vi "pp2_stateToDOCode.vi"(11 "State In":T1={"Curr  tr"=0, "Curr (ms)"=0, "Cum (ms)"=0, "Run loop diff"=0, "Curr State"=enum."0 Initialization", "Prev State"=enum."0 Initialization", "Sw1"=FALSE, "Tone Gate"=FALSE, "Stim"=FALSE, "Sw2"=FALSE, "Curr code"=0, "Current Trial"={"Trial Type Number"=1, "Trial Type"=enum."GO", "Trial Weight"=100, "Shock (mA)"=0.3, "Duration (ms)"=0.25, "Type"=enum."04 FM Sweep", "Stim P2"=4000.0, "Stim P3"=0.0, "Stim P4"=0.0, "Stim P1"=2000.0}, "Last tone"=0, "Countdown (ms)"=0, "Next Trial"={"Trial Type Number"=1, "Trial Type"=enum."GO", "Trial Weight"=100, "Shock (mA)"=0.3, "Duration (ms)"=0.25, "Type"=enum."04 FM Sweep", "Stim P2"=4000.0, "Stim P3"=0.0, "Stim P4"=0.0, "Stim P1"=2000.0}, "Current DAQ Digital Out"=0} {"Current DAQ Digital Out" format="%b"; "Next Trial"."Shock (mA)" min=-1.0 max=5.0; "Next Trial"."Trial Weight" step=1; "Next Trial"."Duration (ms)" min=0.0 max=1.0; "Next Trial"."Trial Type Number" min=1 max=256 step=1; "Current Trial"."Shock (mA)" min=-1.0 max=5.0; "Current Trial"."Trial Weight" step=1; "Current Trial"."Duration (ms)" min=0.0 max=1.0; "Current Trial"."Trial Type Number" min=1 max=256 step=1; "Curr code" format="%#.6f"}) -> (3 "DAQ Digital Code":u16 format="%b")   [LabVIEW 2013]
uses:
  pp2_CTL_StateInfo.ctl
  pp2_State.ctl
  pp2_Trial.ctl
  pp2_TrialType.ctl
  labolabo2/waveforms/WFTypes.ctl
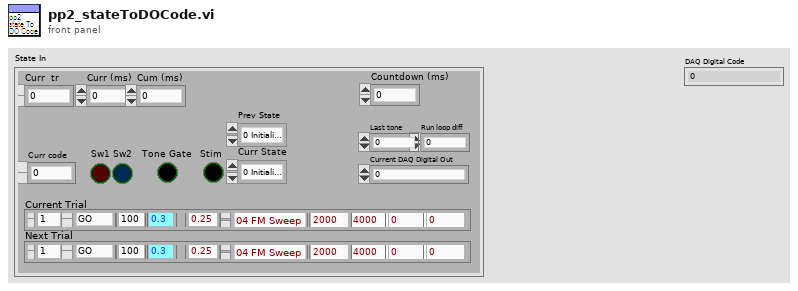
[diagram p1: front panel]
types:
  T1 = typedef "pp2_CTL_StateInfo.ctl" = cluster{"Curr  tr":u16, "Curr (ms)":i64, "Cum (ms)":i64, "Run loop diff":i64, "Curr State":T2, "Prev State":T2, "Sw1":bool, "Tone Gate":bool, "Stim":bool, "Sw2":bool, "Curr code":u8, "Current Trial":T3, "Last tone":i64, "Countdown (ms)":i64, "Next Trial":T3, "Current DAQ Digital Out":u16}
  T2 = typedef "pp2_State.ctl" = enum8{"0 Initialization", "1 Habituation", "2 Load Pre", "3 Wait", "4 Pre/Load Trial", "5 GO Trial", "6 GO Jumped", "7 GO Timeout", "8 NOGO Trial", "9 NOGO Jumped", "10 NOGO Timeout", "11 TEST Trial", "12 TEST Jumped", "13 TEST Timeout", "14 Done"}
  T3 = typedef "pp2_Trial.ctl" = cluster{"Trial Type Number":i16, "Trial Type":T4, "Trial Weight":u32, "Shock (mA)":dbl, "Duration (ms)":dbl, "Type":T5, "Stim P2":dbl, "Stim P3":dbl, "Stim P4":dbl, "Stim P1":dbl}
  T4 = typedef "pp2_TrialType.ctl" = enum16{"OFF", "GO", "NOGO", "TEST"}
  T5 = typedef "WFTypes.ctl" = enum16{"00 NULL", "01 DC", "02 Noise", "03 Pure Tone", "04 FM Sweep"}
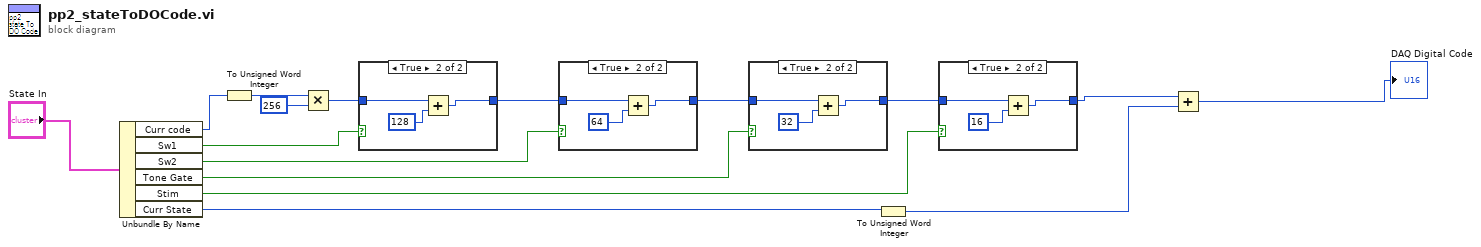
[diagram p0: block diagram]
diagram:
  n1 = Unbundle By Name("State In") -> ("Curr code"=w13:u8, "Sw1"=w14:bool, "Sw2"=w9:bool, "Tone Gate"=w7:bool, "Stim"=w5:bool, "Curr State"=w1:T2)
  n2 = To Unsigned Word Integer(number=w13) -> (unsigned 16bit integer=w12:u16)
  n3 = Multiply(x=w12, y=u16 256) -> (x*y=w11:u16)
  n4 = case shown="True" w14 {
    tunnel: w11 -> [w17 w19]
    tunnel: [w17 w18] -> w10
    frame False {
    }
    frame True {
      n5 = Add(x=w19, y=u16 128 ("Current DAQ Digital Out")) -> (x+y=w18:u16)
    }
  }
  n6 = case shown="True" w9 {
    tunnel: w10 -> [w21 w23]
    tunnel: [w21 w22] -> w8
    frame False {
    }
    frame True {
      n7 = Add(x=w23, y=u16 64 ("Current DAQ Digital Out")) -> (x+y=w22:u16)
    }
  }
  n8 = case shown="True" w7 {
    tunnel: w8 -> [w25 w27]
    tunnel: [w25 w26] -> w6
    frame False {
    }
    frame True {
      n9 = Add(x=w27, y=u16 32 ("Current DAQ Digital Out")) -> (x+y=w26:u16)
    }
  }
  n10 = To Unsigned Word Integer(number=w1) -> (unsigned 16bit integer=w2:u16)
  n11 = case shown="True" w5 {
    tunnel: w6 -> [w29 w31]
    tunnel: [w29 w30] -> w4
    frame False {
    }
    frame True {
      n12 = Add(x=w31, y=u16 16 ("Current DAQ Digital Out")) -> (x+y=w30:u16)
    }
  }
  n13 = Add(x=w4, y=w2) -> (x+y=→"DAQ Digital Code":u16)
